vi "count.vi"(9 "nums":i32[](array[numeric]), 10 "cfg":string, 11 "Map in":map{cluster{string, "nums":i32[]}, u64}(c390)) -> (0 "count":u64, 3 "Map out":map{cluster{string, "nums":i32[]}, u64}(c390))   [LabVIEW 2025, in "d12.lvlib"]
uses:
  d12.lvlib
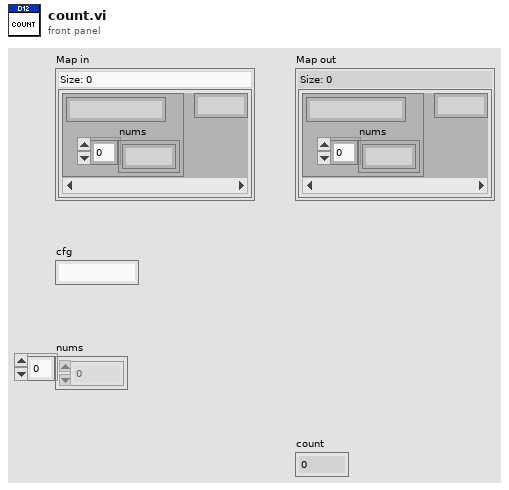
[diagram p1: front panel]
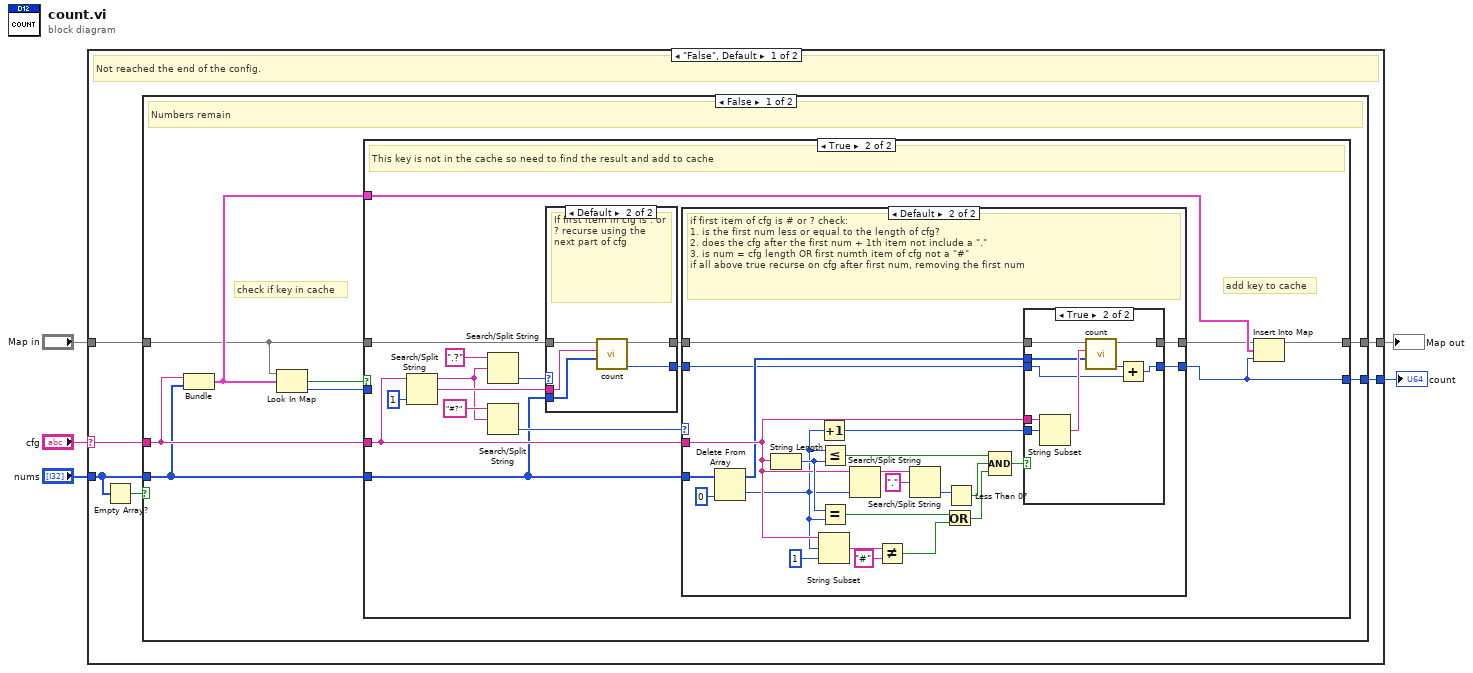
[diagram p0: block diagram]
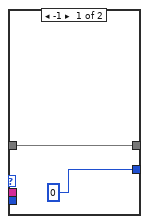
[diagram p5: hidden frame]
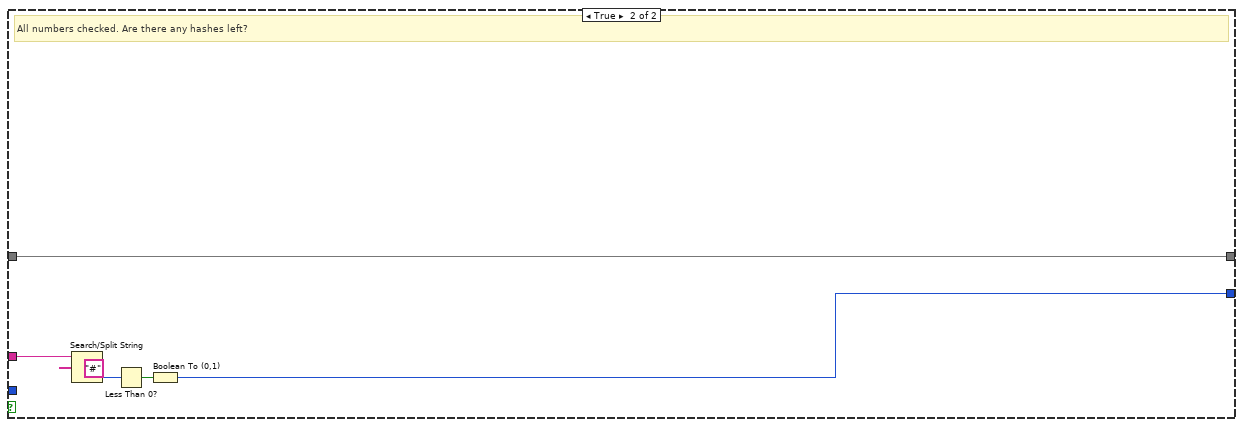
[diagram p6: hidden frame]
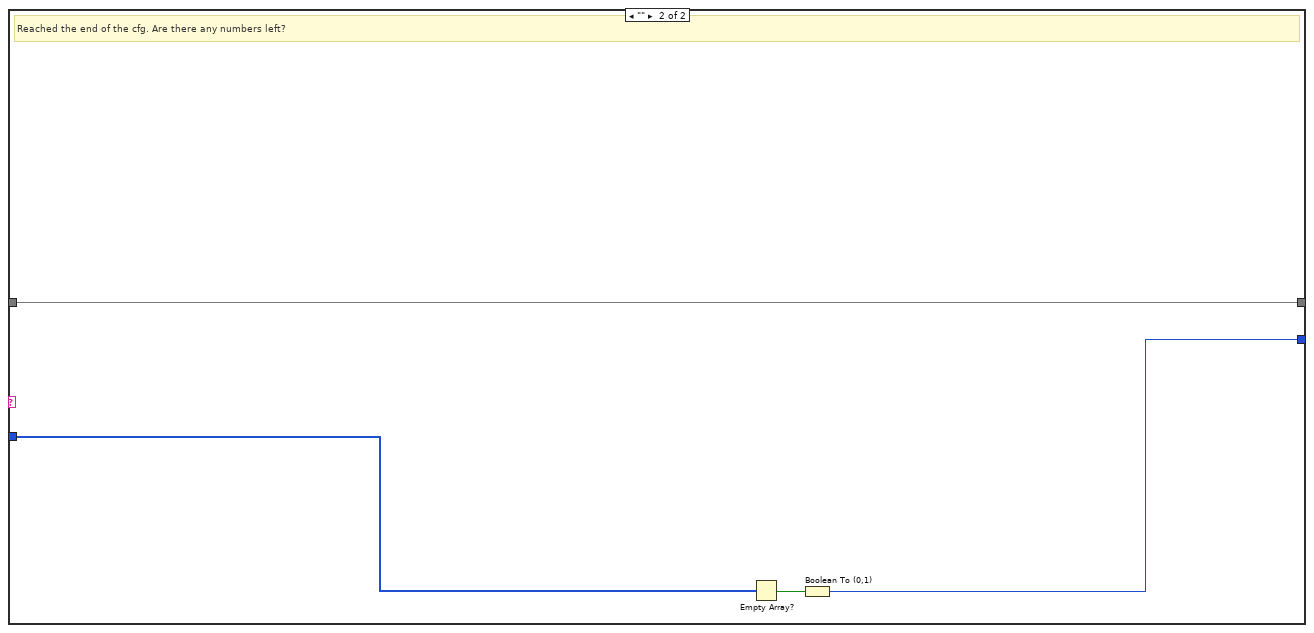
[diagram p7: hidden frame]
diagram:
  n1 = case shown="\"False\", Default" "cfg" {
    selector: "cfg" -> [w9 _]
    tunnel: "nums" -> [w8 w90]
    tunnel: [w10 w88] -> w2
    tunnel: "Map in" -> [w7 w87]
    tunnel: [w6 w87] -> w1
    frame "False", Default {
      # "Not reached the end of the config."
      n2 = Empty Array?(array=w8) -> (empty?=w11:bool)
      n3 = case shown="False" w11 {
        tunnel: w9 -> [w16 w86]
        tunnel: w8 -> [w15 _]
        tunnel: [w17 w82] -> w10
        tunnel: w7 -> [w12 w81]
        tunnel: [w14 w81] -> w6
        frame False {
          # "check if key in cache"
          # "Numbers remain"
          n4 = Bundle(w16, "nums"=w15) -> (w13:cluster{string, "nums":i32[]})  [unwired: 1 in]
          n5 = Look In Map(map=w12, key=w13) -> (key not found?=w19:bool, value=w18:u64)  [unwired: 1 in]
          n6 = case shown="True" w19 {
            tunnel: w18 -> [w21 _]
            tunnel: [w21 w24] -> w17
            tunnel: w12 -> [w20 w28]
            tunnel: w16 -> [_ w29]
            tunnel: w15 -> [_ w25]
            tunnel: [w20 w22] -> w14
            tunnel: w13 -> [_ w26]
            frame False {
              # "Key is in the cache, get the result."
            }
            frame True {
              # "add key to cache"
              # "This key is not in the cache so need to find the result and add to cache"
              n7 = Search/Split String(string=w29, offset (0)=1) -> (substring before match=w31:string, match + rest of string=w34:string)  [unwired: 1 in, 1 out]
              n8 = Search/Split String(string=".?", search string/char (-)=w31) -> (offset of match=w35:i32)  [unwired: 1 in, 2 out]
              n9 = Search/Split String(string="#?", search string/char (-)=w31) -> (offset of match=w30:i32)  [unwired: 1 in, 2 out]
              n10 = case shown="Default" w35 {
                tunnel: w28 -> [w74 w80]
                tunnel: w34 -> [_ w79]
                tunnel: w25 -> [_ w78]
                tunnel: [u64 0 ("count") w77] -> w33
                tunnel: [w74 w76] -> w27
                frame -1 {
                }
                frame Default {
                  # "If first item in cfg is . or ? recurse using the next part of cfg"
                  n11 = call "count.vi"("nums"=w78, "cfg"=w79, "Map in"=w80) -> ("count"=w77:u64, "Map out"=w76:map{cluster{string, "nums":i32[]}, u64})  [unwired: 7 in]
                }
              }
              n12 = case shown="Default" w30 {
                tunnel: w27 -> [w38 w62]
                tunnel: w33 -> [w39 w44]
                tunnel: [w39 w43] -> w24
                tunnel: w29 -> [_ w48]
                tunnel: w25 -> [_ w49]
                tunnel: [w38 w40] -> w23
                frame -1 {
                }
                frame Default {
                  # "if first item of cfg is # or ? check:\n1. is the first num less or equal to the length of cfg?\n2. does the cfg after the first num + 1th item not include a \".\"\n3. is num = cfg length OR first numth item of cfg not a \"#\"\nif all above true recurse on cfg after first num, removing the first num"
                  n13 = Delete From Array(array=w49, index=0) -> (deleted portion=w42:i32, array with subset deleted=w46:i32[])  [unwired: 1 in]
                  n14 = String Length(string=w48) -> (length=w54:i32)
                  n15 = Increment(x=w42) -> (x+1=w41:i32)
                  n16 = String Subset(string=w48, offset (0)=w42, length (rest)=1 ("length (rest)")) -> (substring=w52:string)
                  n17 = Less Or Equal?(x=w42, y=w54) -> (x <= y?=w59:bool)
                  n18 = Equal?(x=w54, y=w42) -> (x = y?=w55:bool)
                  n19 = Search/Split String(string=w48, offset (0)=w42) -> (substring before match=w61:string)  [unwired: 1 in, 2 out]
                  n20 = Not Equal?(x=w52, y="#") -> (x != y?=w50:bool)
                  n21 = Search/Split String(string=w61, search string/char (-)=".") -> (offset of match=w58:i32)  [unwired: 1 in, 2 out]
                  n22 = Or(x=w55, y=w50) -> (x .or. y?=w56:bool)
                  n23 = Less Than 0?(x=w58) -> (x < 0?=w57:bool)
                  n24 = Compound Arithmetic op=AND(w59, w57, w56) -> (w45:bool)
                  n25 = case shown="True" w45 {
                    tunnel: w62 -> [w63 w73]
                    tunnel: w48 -> [_ w72]
                    tunnel: w41 -> [_ w71]
                    tunnel: w46 -> [_ w69]
                    tunnel: w44 -> [w64 w66]
                    tunnel: [w64 w68] -> w43
                    tunnel: [w63 w65] -> w40
                    frame False {
                    }
                    frame True {
                      n26 = String Subset(string=w72, offset (0)=w71) -> (substring=w70:string)  [unwired: 1 in]
                      n27 = call "count.vi"("nums"=w69, "cfg"=w70, "Map in"=w73) -> ("count"=w67:u64, "Map out"=w65:map{cluster{string, "nums":i32[]}, u64})  [unwired: 7 in]
                      n28 = Add(x=w67, y=w66) -> (x+y=w68:u64)
                    }
                  }
                }
              }
              n29 = Insert Into Map(map in=w23, key=w26, value=w24) -> (map out=w22:map{cluster{string, "nums":i32[]}, u64})  [unwired: 2 out]
            }
          }
        }
        frame True {
          # "All numbers checked. Are there any hashes left?"
          n30 = Search/Split String(string=w86, search string/char (-)="#") -> (offset of match=w84:i32)  [unwired: 1 in, 2 out]
          n31 = Less Than 0?(x=w84) -> (x < 0?=w83:bool)
          n32 = Boolean To (0,1)(Boolean=w83) -> (0, 1=w82:i16)
        }
      }
    }
    frame "" {
      # "Reached the end of the cfg. Are there any numbers left?"
      n33 = Empty Array?(array=w90) -> (empty?=w89:bool)
      n34 = Boolean To (0,1)(Boolean=w89) -> (0, 1=w88:i16)
    }
  }
  "count" <- w2
  "Map out" <- w1
